vi "SplitTIFF.vi"() -> ()   [LabVIEW 2011]
uses:
  Library/tiff/TiffModules/AddTiffPage_U16_text_res.vi
panel:
  out "out-name":string
  in  "Split":i32=192
  in  "Clear string":bool=TRUE
  in  "Output type":u16(ring)=257 items=["Big-Endian"=0, "Native"=1, "Little-Endian"=2, "BigTiff-Big-Endian"=256, "Bigtiff,Native"=257, "Biftiff,Littleendian"=258]
  in  "Inputfile":path=path "C:/temp/20240508-Beads/I39/I39_B1_Raw.tif"
  in  "Stop at read offset:":u64=429496729500
  out "AfterDIRoffset":u64 format="%09d"
  out "Input-page":i32
  out "string":string
  out "xy-resolution":cluster{"x":dbl, "y":dbl}
  out "In":u16[][](graph)
  # "select tiff file\nenter split, it will split if modulo=0\nrun\nnew name with _part0.tif\nstops at end or max tiff-offset"
  # "0..n-1 in first file"
  # "<<4294967295 for std Tiff"
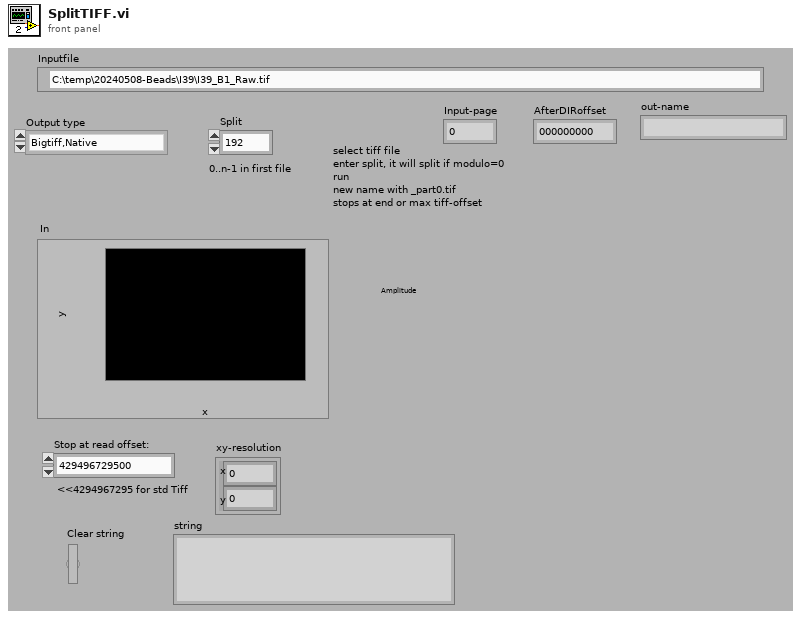
[diagram p1: front panel]
types:
  T1 = cluster{"Tiff refnum":refnum<file>, "BigTiff,Endian":u16}
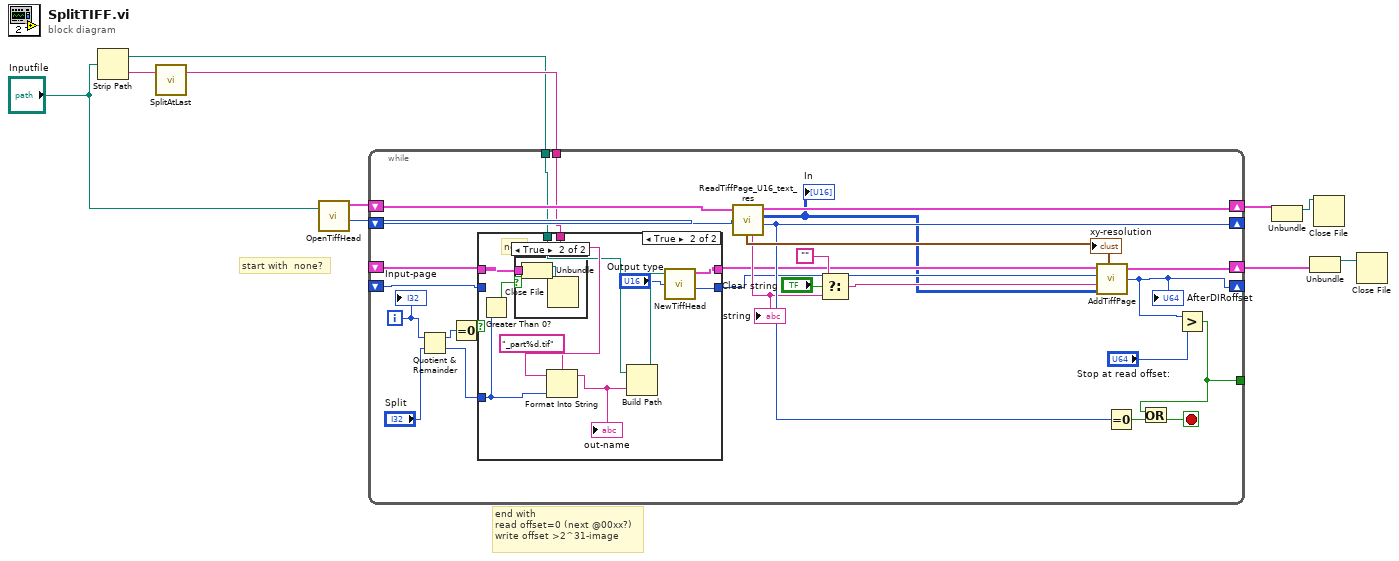
[diagram p0: block diagram]
diagram:
  # "start with  none?"
  # "end with \nread offset=0 (next @00xx?)\nwrite offset >2^31-image"
  n1 = Strip Path(path="Inputfile") -> (stripped path=w1:path, name=w8:string)
  n2 = call "SplitAtLast.vi"("In-String"=w8) -> ("Front (default)"=w2:string)  [unwired: 1 in, 1 out]
  n3 = call "OpenTiffHead.vi"("file path"="Inputfile") -> ("TIFF file"=w7:T1, "first Diroffset"=w6:u64)  [unwired: 2 in, 1 out]
  n4 = while {
    shift-right: [w32] -> w5
    shift-left: w7 -> [w35]
    shift-right: [w37] -> w10
    shift-left: _ -> [w19]
    shift-right: [w31] -> _
    shift-left: w6 -> [w34]
    shift-right: [w12] -> _
    shift-left: _ -> [w16]
    tunnel: [w28] -> _
    tunnel: w2 -> [w14]
    tunnel: w1 -> [w13]
    i -> [w22]
    stop <- w29 stop-if-true
    n5 = Quotient & Remainder(x=w22, y="Split") -> (x-y*floor(x/y)=w21:i32, floor(x/y)=w15:i32)
    n6 = Equal To 0?(x=w21) -> (x = 0?=w20:bool)
    n7 = case shown="True" w20 {
      tunnel: w19 -> [w39 w50]
      tunnel: [w39 w49] -> w18
      tunnel: w16 -> [w38 _]
      tunnel: [w38 w48] -> w17
      tunnel: w15 -> [_ w40]
      tunnel: w14 -> [_ w47]
      tunnel: w13 -> [_ w44]
      frame False {
      }
      frame True {
        # "new"
        n8 = Greater Than 0?(x=w40) -> (x > 0?=w41:bool)
        n9 = case shown="True" w41 {
          tunnel: w50 -> [_ w51]
          frame False {
          }
          frame True {
            n10 = Unbundle(w51) -> ("Tiff refnum"=w52:refnum<file>)  [unwired: 1 out]
            n11 = Close File(refnum=w52) -> ()  [unwired: 1 in, 2 out]
          }
        }
        n12 = Format Into String(format string="_part%d.tif", initial string=w47, w40) -> (resulting string=w45:string)  [unwired: 1 in, 1 out]
        "out-name" <- w45
        n13 = Build Path(base path=w44, name or relative path=w45) -> (appended path=w43:path)
        n14 = call "NewTiffHead.vi"("file path"=w43, "BigTiff,Endian"="Output type") -> ("TIFF file"=w49:T1, "Place for first IFD (8,eof-position)"=w48:u64)  [unwired: 2 in, 1 out]
      }
    }
    n15 = call "ReadTiffPage_U16_text_res.vi"("TIFF file"=w35, "IFDoffset"=w34) -> ("Pixelsize [µm]"=w33:cluster{"x":dbl, "y":dbl}, "TIFF file out"=w32:T1, "16-bit pixmap"=w11:u16[][], "string"=w26:string, "Next offset"=w31:i64)  [unwired: 3 in, 1 out]
    "In" <- w11
    "xy-resolution" <- w33
    "string" <- w26
    n16 = Select(t="", s="Clear string", f=w26) -> (s? t:f=w27:string)
    n17 = call-poly "AddTiffPage.vi"("TIFF file"=w18, "After last DIROffset"=w17, "Text"=w27, "16-bit pixmap x, y"=w11, "Pixelsize [µm]"=w33) -> ("TIFF file"=w37:T1, "AfterDIRoffset"=w12:u64)  [unwired: 1 out]
    "AfterDIRoffset" <- w12
    n18 = Equal To 0?(x=w31) -> (x = 0?=w36:bool)
    n19 = Greater?(x=w12, y="Stop at read offset:") -> (0:w28:bool)
    n20 = Or(x=w28, y=w36) -> (x .or. y?=w29:bool)
    "Input-page" <- w22
  }
  n21 = Unbundle(w5) -> ("Tiff refnum"=w4:refnum<file>)  [unwired: 1 out]
  n22 = Unbundle(w10) -> ("Tiff refnum"=w9:refnum<file>)  [unwired: 1 out]
  n23 = Close File(refnum=w4) -> ()  [unwired: 1 in, 2 out]
  n24 = Close File(refnum=w9) -> ()  [unwired: 1 in, 2 out]
